vi "IsHotGoalDB.vi"(8 "error in":errorcluster, 9 "DBHot?":string="Boolean", 10 "DBFinished?":string="Boolean", 11 "DBStart":string="Boolean") -> (0 "error out":errorcluster, 2 "Hot?":bool)   [LabVIEW 2013]
doc: "IsHotGoalDB determines whether or not the goal is hot. Image processing is done on the laptop (through the DB).\n-DBStart: the name of the DB boolean control that starts image processing. IsHotGoalDB writes to this to signal the DB to start.\n-DBFinished?: the name of the DB boolean indicator that indicates when the DB is done processing.\n-DBHot?: the name of the DB boolean indicator that indicates whether the goal is hot."
panel:
  in  "milliseconds to wait":u32=20
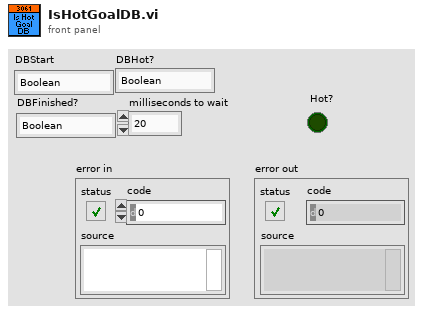
[diagram p1: front panel]
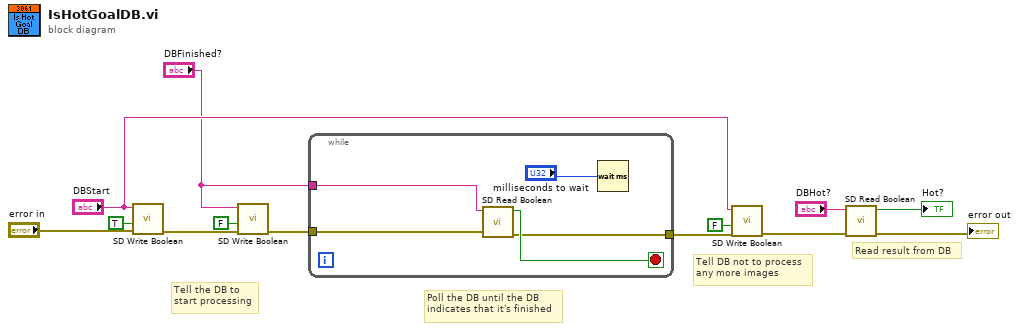
[diagram p0: block diagram]
diagram:
  # "Tell DB not to process\nany more images"
  # "Read result from DB"
  # "Poll the DB until the DB\nindicates that it's finished"
  # "Tell the DB to\nstart processing"
  n1 = call <vilib>:"SD Write Boolean.vi"("error in"="error in", "Boolean"=TRUE, "Name"="DBStart") -> ("error out"=w4:errorcluster)  [unwired: 7 in, 1 out]
  n2 = call <vilib>:"SD Write Boolean.vi"("error in"=w4, "Boolean"=FALSE, "Name"="DBFinished?") -> ("error out"=w3:errorcluster)  [unwired: 7 in, 1 out]
  n3 = while {
    tunnel: w3 -> [w18]
    tunnel: [w16] -> w7
    tunnel: "DBFinished?" -> [w14]
    stop <- w17 stop-if-true
    n4 = call <vilib>:"SD Read Boolean.vi"("error in"=w18, "Name"=w14) -> ("error out"=w16:errorcluster, "Boolean"=w17:bool)  [unwired: 7 in, 1 out]
    n5 = Wait (ms)(milliseconds to wait="milliseconds to wait") -> ()  [unwired: 1 out]
  }
  n6 = call <vilib>:"SD Write Boolean.vi"("error in"=w7, "Boolean"=FALSE, "Name"="DBStart") -> ("error out"=w6:errorcluster)  [unwired: 7 in, 1 out]
  n7 = call <vilib>:"SD Read Boolean.vi"("error in"=w6, "Name"="DBHot?") -> ("error out"=→"error out":errorcluster, "Boolean"=→"Hot?":bool)  [unwired: 7 in, 1 out]
